vi "Obtain Msg Q DVR.vi"(10 "Msg Q DVR Alias":string) -> (0 "error out":errorcluster, 2 "Msg Q DVR":refnum<data-value>)   [LabVIEW 2021, in "LVCAM.lvlib"]
uses:
  LVCAM.lvlib
  Msg Strategy/Msg Strategy.lvclass
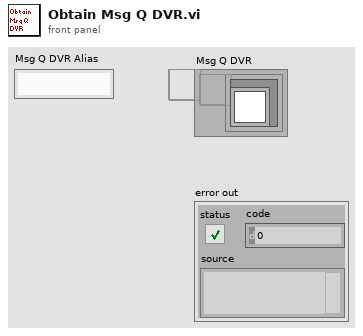
[diagram p1: front panel]
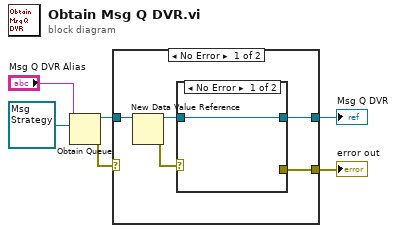
[diagram p0: block diagram]
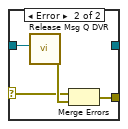
[diagram p2: hidden frame]
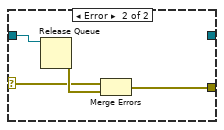
[diagram p3: hidden frame]
diagram:
  n1 = Obtain Queue(name (unnamed)="Msg Q DVR Alias", element data type=refnum<class "Msg Strategy.lvclass"> refnum ("Artifex Actor Model.lvlib:Msg.lvclass")) -> (queue out=w3:refnum<queue>, error out=w6:errorcluster)  [unwired: 3 in, 1 out]
  n2 = case shown="No Error" w6 {
    selector: w6 -> [_ w17]
    tunnel: w3 -> [w11 w20]
    tunnel: [w8 _] -> w2
    tunnel: [w9 w19] -> w1
    frame No Error {
      n3 = New Data Value Reference(data value=w11) -> (data value reference=w7:refnum<data-value>, error out=w10:errorcluster)  [unwired: 1 in]
      n4 = case shown="No Error" w10 {
        selector: w10 -> [_ w13]
        tunnel: [_ w15] -> w9
        tunnel: [w12 _] -> w8
        tunnel: w7 -> [w12 w16]
        frame No Error {
        }
        frame Error {
          n5 = call "Release Msg Q DVR.vi"("Msg Q DVR"=w16) -> ("error out"=w14:errorcluster)  [unwired: 10 in]
          n6 = Merge Errors(w13, w14) -> (w15:errorcluster)
        }
      }
    }
    frame Error {
      n7 = Release Queue(queue=w20) -> (error out=w18:errorcluster)  [unwired: 2 in, 2 out]
      n8 = Merge Errors(w17, w18) -> (w19:errorcluster)
    }
  }
  "Msg Q DVR" <- w2
  "error out" <- w1
